vi "charge_salairial.vi"() -> ()   [LabVIEW 2024]
panel:
  out "Charge salairial":dbl
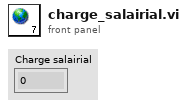
[diagram p1: front panel]
diagram:
